vi "Clean.vi"(0 "NI Build Specification_LV in":refnum<class "NI Build Specification_LV.lvclass">) -> (4 "NI Build Specification_LV out":refnum<class "NI Build Specification_LV.lvclass">)   [LabVIEW 2017, in "CL_G3_VIComponentBuilder.lvlib" / "NI Build Specification_LV.lvclass"]
doc: "Removes this export from the build machine.\n <MustCallParent>The parent creates various files therefore the parent's clean method must be called to clean up those files.</MustCallParent>"
uses:
  NI Build Specification_LV.lvclass
  C:/Tool Chain Support/Software Module Builder/Source/Exports/Exports/Export.lvclass
  Exports/Export.lvclass/Export.ctl
  Exports/Accessors/Read Component Export Dir.vi
  Exports/Accessors/Read Export Operation Errors.vi
  Exports/Accessors/Write Export Operation Errors.vi
  Exports/Export.lvclass
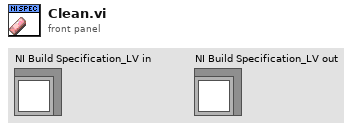
[diagram p1: front panel]
types:
  T1 = cluster{"Error State":errorcluster, "Build Spec":refnum<class "NI Build Specification_LV.lvclass">}
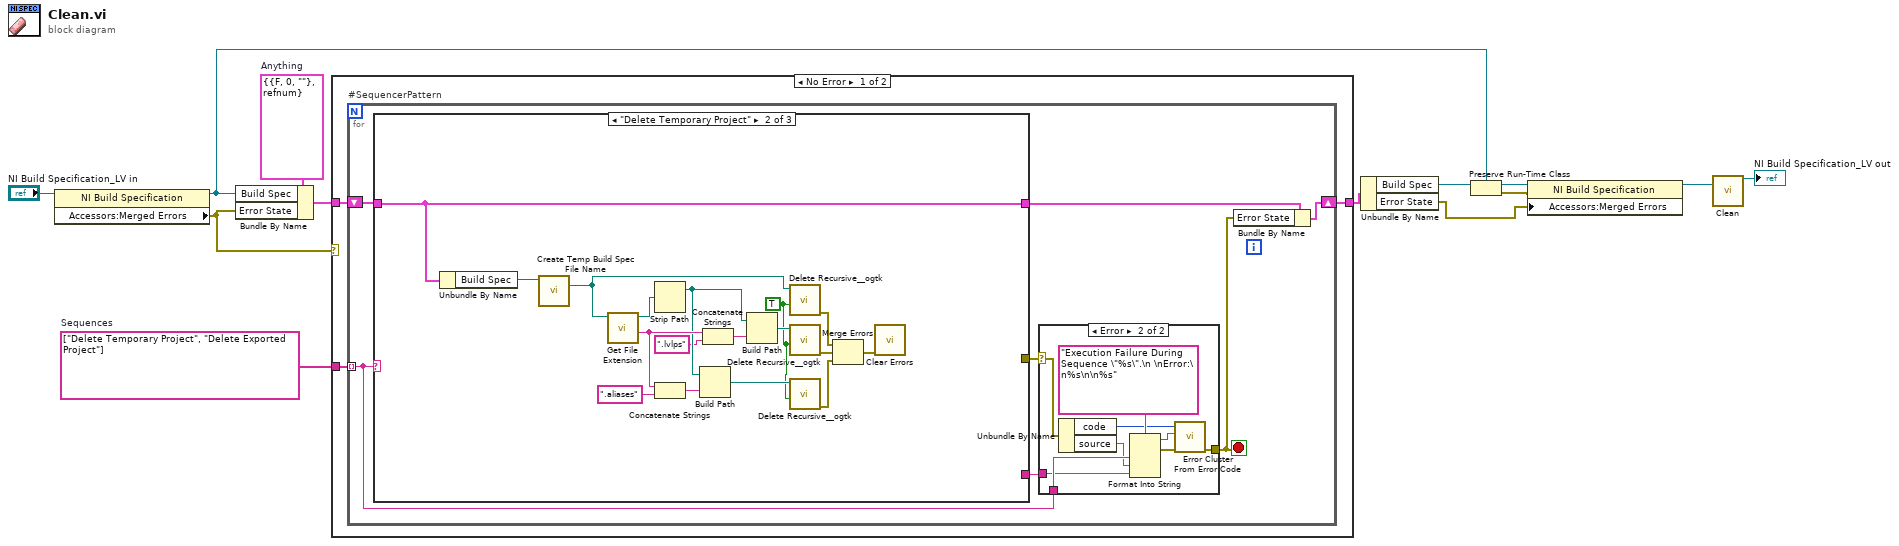
[diagram p0: block diagram]
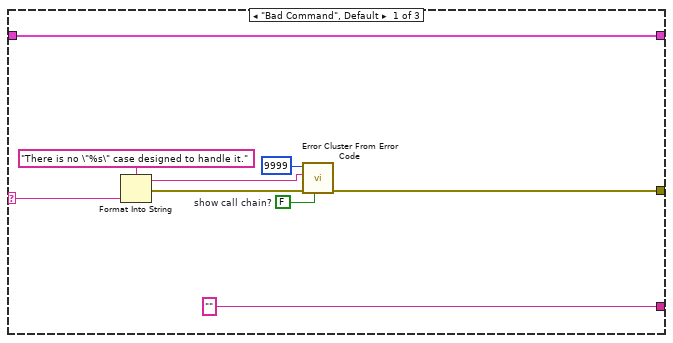
[diagram p3: hidden frame]
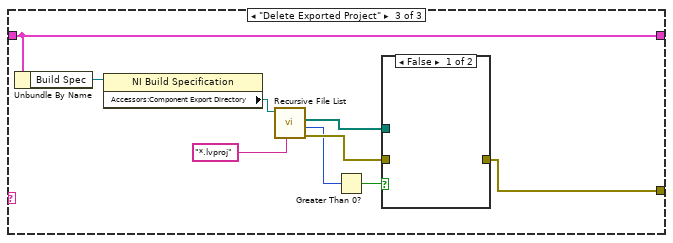
[diagram p4: hidden frame]
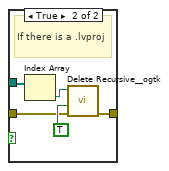
[diagram p5: hidden frame]
diagram:
  w12 = T1 {"Error State"={"status"=FALSE, "code"=0, "source"=""}, "Build Spec"=refnum}  # Anything
  w10 = string[] ["Delete Temporary Project", "Delete Exported Project"]  # Sequences
  n1 = property class="NI Build Specification"(reference="NI Build Specification_LV in") -> (reference out=w4:refnum<class "NI Build Specification_LV.lvclass">, "Accessors:Merged Errors"=w9:errorcluster)  [unwired: 1 in, 1 out]
  n2 = Bundle By Name(cluster=w12, "Build Spec"=w4, "Error State"=w9) -> (w8:T1)
  n3 = case shown="No Error" w9 {
    tunnel: w10 -> [w16 _]
    tunnel: w8 -> [w15 w74]
    tunnel: [w14 w74] -> w11
    frame No Error {
      n4 = for "#SequencerPattern" {
        tunnel: w16 -> [w19] mode=indexing
        shift-right: [w22] -> w14
        shift-left: w15 -> [w23]
        stop <- w17 stop-if-true
        n5 = case shown="\"Delete Temporary Project\"" w19 {
          selector: w19 -> [w39 _ _]
          tunnel: w23 -> [w42 w45 w63]
          tunnel: [w42 w45 w63] -> w21
          tunnel: [w38 _ w60] -> w20
          tunnel: ["" ("Accessors:Name") _ _] -> w18
          frame "Bad Command", Default {
            w34 = FALSE  # show call chain?
            n6 = Format Into String(format string="There is no \"%s\" case designed to handle it.", w39) -> (resulting string=w37:string, error out=w35:errorcluster)  [unwired: 2 in]
            n7 = call <vilib>:"Error Cluster From Error Code.vi"("show call chain? (False)"=w34, "error in (no error)"=w35, "error message (\"\")"=w37, "error code (0)"=9999 ("Error Code")) -> ("error out"=w38:errorcluster)  [unwired: 5 in]
          }
          frame "Delete Temporary Project" {
            w46 = TRUE ("Ignore Read-Only? (FALSE)")
            n8 = Unbundle By Name(w45) -> ("Build Spec"=w44:refnum<class "NI Build Specification_LV.lvclass">)
            n9 = call "Create Temp Build Spec File Name.vi"("Export"=w44) -> ("Temporary build spec Path"=w43:path)  [unwired: 12 in, 2 out]
            n10 = call <vilib>:"Get File Extension.vi"("file"=w43) -> ("filename without extension"=w50:string, "dup file"=w58:path)  [unwired: 6 in, 3 out]
            n11 = Strip Path(path=w58) -> (stripped path=w49:path)  [unwired: 1 out]
            n12 = Concatenate Strings(w50, ".aliases" ("string")) -> (w55:string)
            n13 = Build Path(base path=w49, name or relative path=w55) -> (appended path=w54:path)
            n14 = Concatenate Strings(w50, ".lvlps" ("string")) -> (w57:string)
            n15 = Build Path(base path=w49, name or relative path=w57) -> (appended path=w56:path)
            n16 = call <userlib>:"Delete Recursive__ogtk.vi"("Ignore Read-Only? (FALSE)"=w46, "Path"=w43) -> ("error out"=w52:errorcluster)  [unwired: 8 in, 1 out]
            n17 = call <userlib>:"Delete Recursive__ogtk.vi"("Ignore Read-Only? (FALSE)"=w46, "Path"=w56) -> ("error out"=w53:errorcluster)  [unwired: 8 in, 1 out]
            n18 = call <userlib>:"Delete Recursive__ogtk.vi"("Ignore Read-Only? (FALSE)"=w46, "Path"=w54) -> ("error out"=w59:errorcluster)  [unwired: 8 in, 1 out]
            n19 = Merge Errors(w52, w53, w59) -> (w51:errorcluster)
            n20 = call <vilib>:"Clear Errors.vi"("error in (no error)"=w51) -> ()  [unwired: 5 in, 2 out]
          }
          frame "Delete Exported Project" {
            n21 = Unbundle By Name(w63) -> ("Build Spec"=w62:refnum<class "NI Build Specification_LV.lvclass">)
            n22 = property class="NI Build Specification"(reference=w62) -> ("Accessors:Component Export Directory"=w61:path)  [unwired: 1 in, 2 out]
            n23 = call <vilib>:"Recursive File List.vi"("pattern"="*.lvproj", "Folder Path"=w61) -> ("error out"=w68:errorcluster, "Number of Files"=w65:i32, "All Files in Dir"=w67:path[])  [unwired: 5 in, 2 out]
            n24 = Greater Than 0?(x=w65) -> (x > 0?=w66:bool)
            n25 = case shown="False" w66 {
              tunnel: w67 -> [_ w73]
              tunnel: w68 -> [_ w70]
              tunnel: [_ w69] -> w60
              frame False {
              }
              frame True {
                # "If there is a .lvproj"
                n26 = Index Array(array=w73) -> (element=w72:path)  [unwired: 1 in]
                n27 = call <userlib>:"Delete Recursive__ogtk.vi"("error in (no error)"=w70, "Ignore Read-Only? (FALSE)"=TRUE, "Path"=w72) -> ("error out"=w69:errorcluster)  [unwired: 7 in, 1 out]
              }
            }
          }
        }
        n28 = case shown="Error" w20 {
          selector: w20 -> [w24 w29]
          tunnel: [w24 w33] -> w17
          tunnel: w19 -> [_ w31]
          tunnel: w18 -> [_ w27]
          frame No Error {
          }
          frame Error {
            n29 = Unbundle By Name(w29) -> ("code"=w25:i32, "source"=w28:string)
            n30 = Format Into String(format string="Execution Failure During Sequence \"%s\".\n \nError:\n%s\n\n%s" ("error message (\"\")"), w31, w28, w27) -> (resulting string=w32:string, error out=w26:errorcluster)  [unwired: 2 in]
            n31 = call <vilib>:"Error Cluster From Error Code.vi"("error in (no error)"=w26, "error message (\"\")"=w32, "error code (0)"=w25) -> ("error out"=w33:errorcluster)  [unwired: 6 in]
          }
        }
        n32 = Bundle By Name(cluster=w21, "Error State"=w17) -> (w22:T1)
      }
    }
    frame Error {
    }
  }
  n33 = Unbundle By Name(w11) -> ("Build Spec"=w3:refnum<class "NI Build Specification_LV.lvclass">, "Error State"=w7:errorcluster)
  n34 = Preserve Run-Time Class(object in=w3, 2:w4) -> (object out=w2:refnum<class "NI Build Specification_LV.lvclass">, error out=w1:errorcluster)  [unwired: 1 in]
  n35 = property class="NI Build Specification"(reference=w2, error in=w1, "Accessors:Merged Errors"=w7) -> (reference out=w6:refnum<class "NI Build Specification_LV.lvclass">)  [unwired: 1 out]
  n36 = call-parent "Clean.vi"("Export in"=w6) -> ("Export out"=→"NI Build Specification_LV out":refnum<class "NI Build Specification_LV.lvclass">)  [unwired: 14 in]
